vi "Write configuration.vi"(8 "error in (no error)":errorcluster, 10 "configuration":refnum<class "CEF_serializable configuration.lvclass">, 11 "Abstract Digitizer":refnum<class "Digitizer Instrument.lvclass">) -> (0 "error out":errorcluster, 3 "Abstract Digitizer out":refnum<class "Digitizer Instrument.lvclass">)   [LabVIEW 2025, in "Digitizer.lvlib" / "Digitizer Instrument.lvclass"]
uses:
  Digitizer Instrument.lvclass
  Users/Public/Documents/Sandia National Labs/TSS Plugin/CEF.lvlibp/serializable configuration/CEF_serializable configuration.lvclass
  Digitizer configuration/Digitizer configuration.lvclass
  Digitizer Instrument.lvclass/Digitizer Instrument.ctl
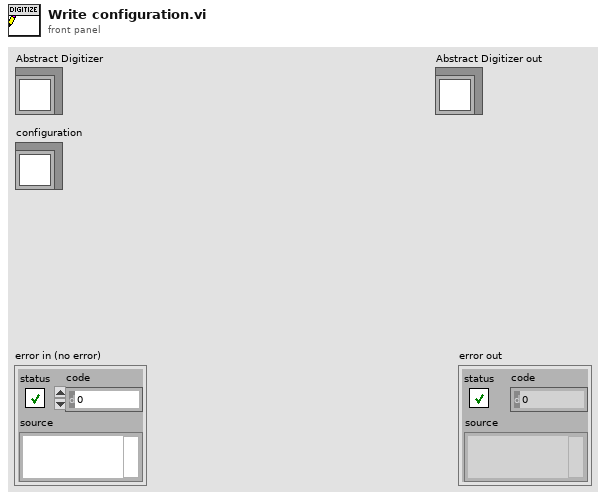
[diagram p1: front panel]
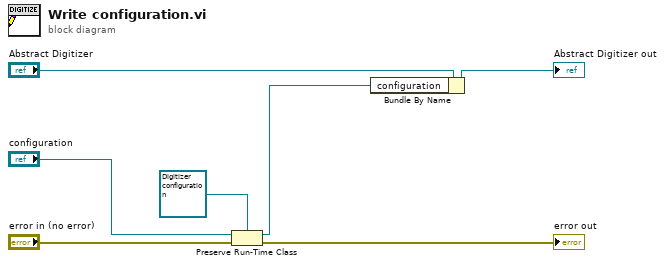
[diagram p0: block diagram]
diagram:
  n1 = Preserve Run-Time Class(object in="configuration", error in="error in (no error)", 2:refnum<class "Digitizer configuration.lvclass"> refnum ("Digitizer.lvlib:Digitizer configuration.lvclass")) -> (object out=w4:refnum<class "Digitizer configuration.lvclass">, error out=→"error out":errorcluster)
  n2 = Bundle By Name(cluster="Abstract Digitizer", "configuration"=w4) -> (→"Abstract Digitizer out":refnum<class "Digitizer Instrument.lvclass">)
